vi "布尔取反 (子VI).vi"(10 "Signal":bool, 11 "Enable¿":bool) -> (3 "Output":bool)   [LabVIEW 2017]
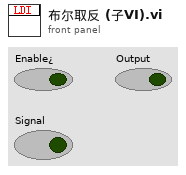
[diagram p1: front panel]
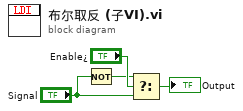
[diagram p0: block diagram]
diagram:
  n1 = Not(x="Signal") -> (.not. x?=w1:bool)
  n2 = Select(t=w1, s="Enable¿", f="Signal") -> (s? t:f=→"Output":bool)
